vi "Untitled 2.vi"() -> ()   [LabVIEW 2017]
panel:
  out "length":i32
  in  "Please add path":path
  out "prompt (Open existing file)":string
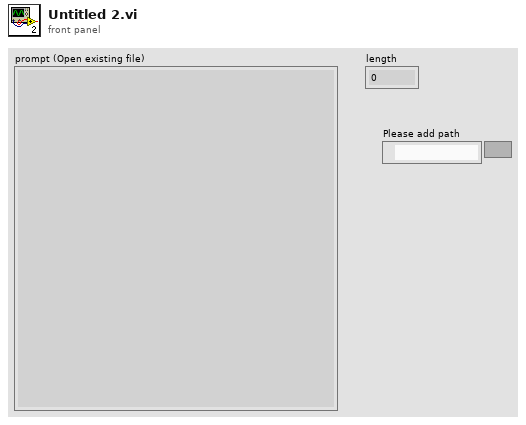
[diagram p1: front panel]
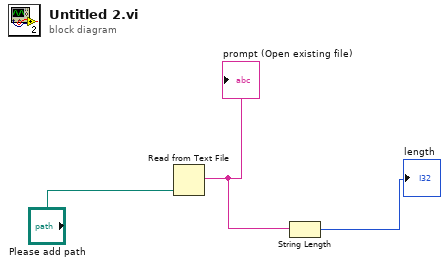
[diagram p0: block diagram]
diagram:
  n1 = Read from Text File(file (use dialog)="Please add path") -> (text=w2:string)  [unwired: 3 in, 3 out]
  "prompt (Open existing file)" <- w2
  n2 = String Length(string=w2) -> (length=→"length":i32)
